vi "Convert Position Real to Target.vi"(5 "PPR":dbl=1024.0 format="%#_13g", 7 "Zero Value":dbl, 11 "Real Position":dbl) -> (2 "Offset Out":dbl, 3 "Position (0-1)":dbl)   [LabVIEW 2023, in "SwerveDrive_ACT_ts.lvlib"]
uses:
  SwerveDrive_ACT_ts.lvlib
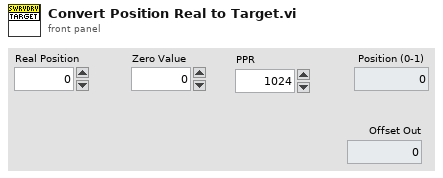
[diagram p1: front panel]
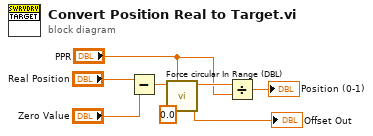
[diagram p0: block diagram]
diagram:
  n1 = Subtract(x="Real Position", y="Zero Value") -> (x-y=w8:dbl)
  n2 = call "Force circular In Range (DBL).vi"("Max"="PPR", "Min"=0.0 ("y"), "Value"=w8) -> ("Offset Out"=→"Offset Out":dbl, "Value Out"=w7:dbl)  [unwired: 7 in]
  n3 = Divide(x=w7, y="PPR") -> (x/y=→"Position (0-1)":dbl)
